vi "AlliGator Test FLI Dataset [All] Loading.vi"(8 "error in (no error)":errorcluster, 11 "AlliGator Q in":refnum<queue>) -> (0 "error out":errorcluster, 3 "AlliGator Q out":refnum<queue>)   [LabVIEW 2021, in "AlliGator Files Tests.lvlib"]
uses:
  AlliGator Files Tests.lvlib
  AlliGator Q Element.ctl
  AlliGator Q Event.ctl
  AlliGator Action Engine.lvlib
panel:
  # "see the AlliGator License on the block diagram (Ctrl+E or Window:Show Block Diagram)"
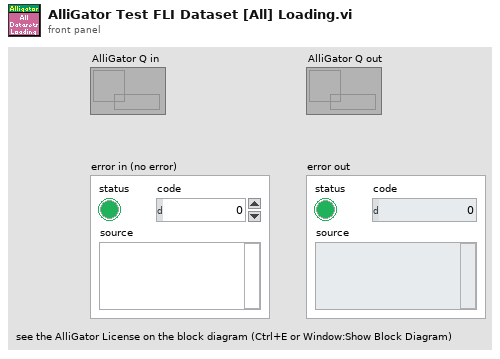
[diagram p1: front panel]
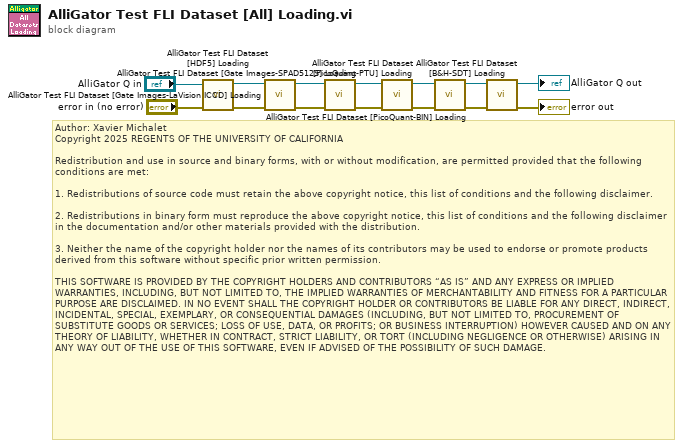
[diagram p0: block diagram]
diagram:
  # "Author: Xavier Michalet\nCopyright 2025 REGENTS OF THE UNIVERSITY OF CALIFORNIA\n\nRedistribution and use in source and binary forms, with or without modification, are permitted provided that the following conditions are met:\n\n1. Redistributions of source code must retain the above copyright notice, this list of conditions and the following disclaimer.\n\n2. Redistributions in binary form must reproduce the above copyright notice, this list of conditions and the following disclaimer in the documentation and/or other materials provided with the distribution.\n\n3. Neither the name of the copyright holder nor the names of its contributors may be used to endorse or promote products derived from this software without specific prior written permission.\n\nTHIS SOFTWARE IS PROVIDED BY THE COPYRIGHT HOLDERS AND CONTRIBUTORS “AS IS” AND ANY EXPRESS OR IMPLIED WARRANTIES, INCLUDING, BUT NOT LIMITED TO, THE IMPLIED WARRANTIES OF MERCHANTABILITY AND FITNESS FOR A PARTICULAR PURPOSE ARE DISCLAIMED. IN NO EVENT SHALL THE COPYRIGHT HOLDER OR CONTRIBUTORS BE LIABLE FOR ANY DIRECT, INDIRECT, INCIDENTAL, SPECIAL, EXEMPLARY, OR CONSEQUENTIAL DAMAGES (INCLUDING, BUT NOT LIMITED TO, PROCUREMENT OF SUBSTITUTE GOODS OR SERVICES; LOSS OF USE, DATA, OR PROFITS; OR BUSINESS INTERRUPTION) HOWEVER CAUSED AND ON ANY THEORY OF LIABILITY, WHETHER IN CONTRACT, STRICT LIABILITY, OR TORT (INCLUDING NEGLIGENCE OR OTHERWISE) ARISING IN ANY WAY OUT OF THE USE OF THIS SOFTWARE, EVEN IF ADVISED OF THE POSSIBILITY OF SUCH DAMAGE."
  n1 = call "AlliGator Test FLI Dataset [HDF5] Loading.vi"("Error In"="error in (no error)", "AlliGator Q in"="AlliGator Q in") -> ("Error Out"=w10:errorcluster, "AlliGator Q out"=w12:refnum<queue>)  [unwired: 8 in]
  n2 = call "AlliGator Test FLI Dataset [Gate Images-LaVision ICCD] Loading.vi"("Error In"=w10, "AlliGator Q in"=w12) -> ("Error Out"=w8:errorcluster, "AlliGator Q out"=w9:refnum<queue>)  [unwired: 8 in]
  n3 = call "AlliGator Test FLI Dataset [Gate Images-SPAD512S] Loading.vi"("Error In"=w8, "AlliGator Q in"=w9) -> ("Error Out"=w1:errorcluster, "AlliGator Q out"=w3:refnum<queue>)  [unwired: 8 in]
  n4 = call "AlliGator Test FLI Dataset [PicoQuant-PTU] Loading.vi"("Error In"=w1, "AlliGator Q in"=w3) -> ("Error Out"=w2:errorcluster, "AlliGator Q out"=w5:refnum<queue>)  [unwired: 8 in]
  n5 = call "AlliGator Test FLI Dataset [PicoQuant-BIN] Loading.vi"("Error In"=w2, "AlliGator Q in"=w5) -> ("Error Out"=w4:errorcluster, "AlliGator Q out"=w6:refnum<queue>)  [unwired: 8 in]
  n6 = call "AlliGator Test FLI Dataset [B&H-SDT] Loading.vi"("Error In"=w4, "AlliGator Q in"=w6) -> ("Error Out"=→"error out":errorcluster, "AlliGator Q out"=→"AlliGator Q out":refnum<queue>)  [unwired: 8 in]
